vi "to string.vi"(8 "error in":errorcluster, 11 "Modbus Slave configuration in":refnum<class "Modbus Slave configuration.lvclass">) -> (0 "error out":errorcluster, 1 "data":string, 2 "version":string, 3 "Modbus Slave configuration out":refnum<class "Modbus Slave configuration.lvclass">)   [LabVIEW 2013, in "Modbus Slave configuration.lvclass"]
doc: "Provides an interface for saving a module configuration to a file or other serialized data source. It is recommended that all children of this class store data in two sets--data required for its own initialization, and any data required for parent initialization--and that each implementation uses the <b>Call Parent Method</b> primitive to serialize parent information.Platypus Framework 1.0.1.65\nNI Systems Engineering - National Instruments"
uses:
  Modbus Slave configuration.lvclass
  <vilib>/NI/Tag Bus Module Framework/module configuration/TBM module configuration.lvclass
  Modbus Slave configuration.lvclass/Modbus Slave configuration.ctl
  module channel/Modbus Module Channel.lvclass
  <vilib>/NI/Configuration Framework/serializable configuration/NISE_CEF_serializable configuration.lvclass
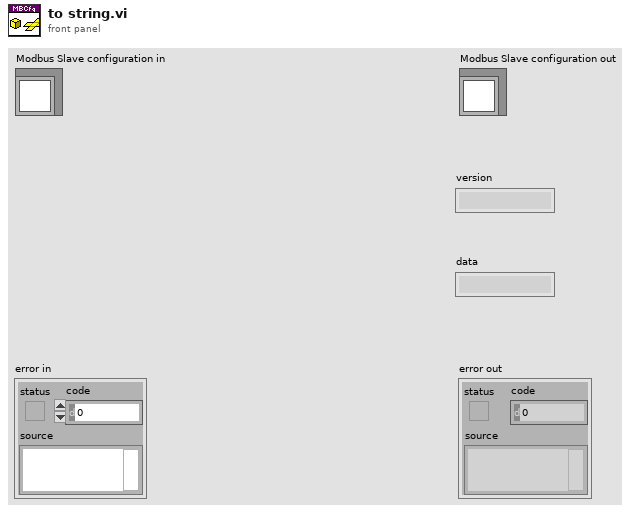
[diagram p1: front panel]
types:
  T1 = typedef "Modbus Slave configuration.lvclass/modbus class.ctl" = enum16{"TCP master", "TCP slave", "serial master", "serial slave"}
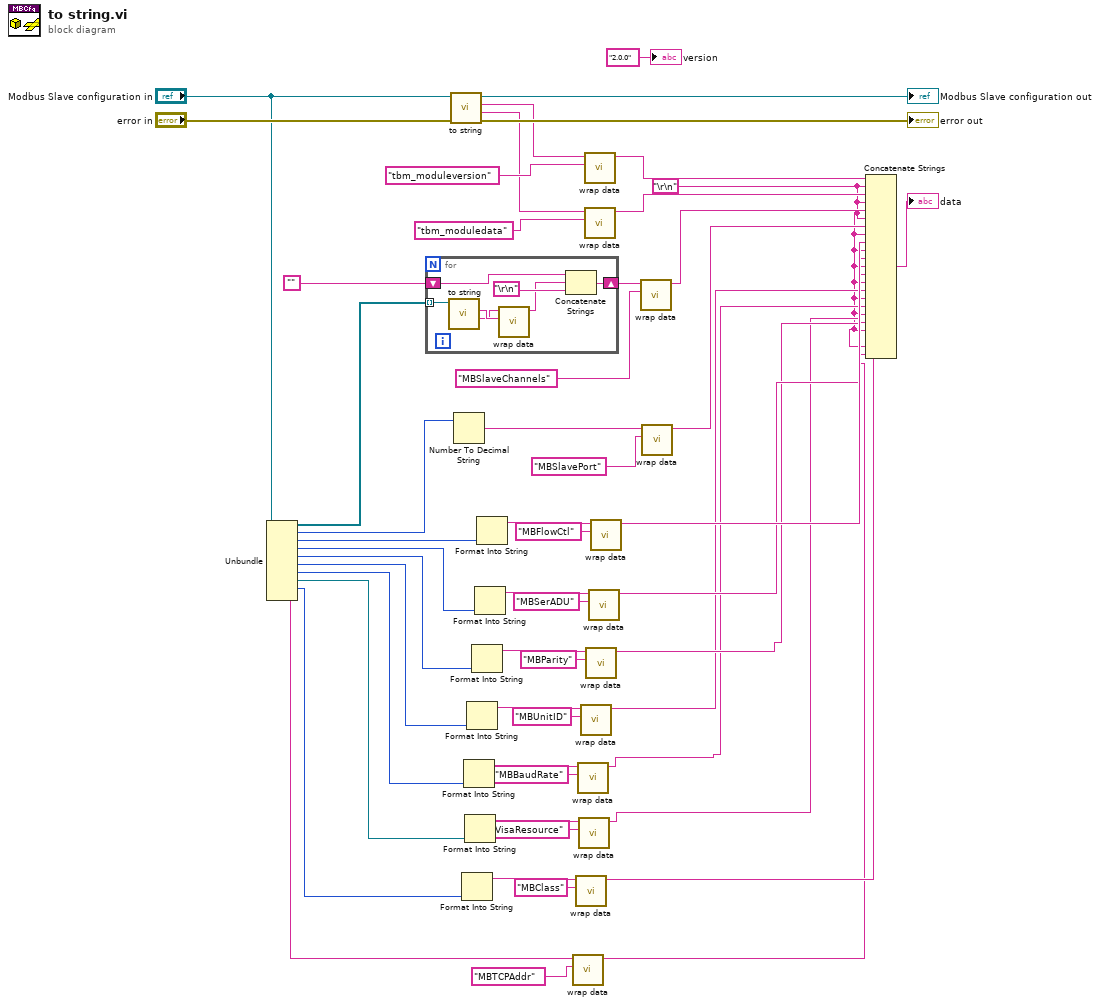
[diagram p0: block diagram]
diagram:
  w4 = "\r\n"
  n1 = Unbundle("Modbus Slave configuration in") -> (w40:refnum<class "Modbus Module Channel.lvclass">[], w35:u16, w31:u16, w17:enum16{"RTU", "ASCII"}, w16:u16, w15:u8, w14:u32, w13:refnum<visa-resource-name>, w12:T1, w3:string)
  n2 = for {
    tunnel: w40 -> [w56] mode=indexing
    shift-right: [w59] -> w38
    shift-left: "" -> [w58]
    n3 = call-dynamic "to string.vi"("channel in"=w56) -> ("channel data"=w54:string, "identifier"=w55:string)  [unwired: 7 in, 2 out]
    n4 = call <vilib>:"wrap data.vi"("identifier"=w55, "data to wrap"=w54) -> ("wrapped data"=w57:string)  [unwired: 9 in]
    n5 = Concatenate Strings(w58, w57, "\r\n") -> (w59:string)
  }
  n6 = call-parent "to string.vi"("error in"="error in", "module configuration in"="Modbus Slave configuration in") -> ("error out"=→"error out":errorcluster, "data"=w45:string, "version"=w46:string, "module configuration out"=→"Modbus Slave configuration out":refnum<class "Modbus Slave configuration.lvclass">)  [unwired: 6 in]
  n7 = Number To Decimal String(number=w35) -> (decimal integer string=w34:string)  [unwired: 1 in]
  n8 = Format Into String(w12) -> (resulting string=w19:string)  [unwired: 3 in, 1 out]
  n9 = Format Into String(w14) -> (resulting string=w24:string)  [unwired: 3 in, 1 out]
  n10 = Format Into String(w13) -> (resulting string=w20:string)  [unwired: 3 in, 1 out]
  n11 = Format Into String(w15) -> (resulting string=w23:string)  [unwired: 3 in, 1 out]
  n12 = Format Into String(w16) -> (resulting string=w27:string)  [unwired: 3 in, 1 out]
  n13 = Format Into String(w17) -> (resulting string=w28:string)  [unwired: 3 in, 1 out]
  n14 = Format Into String(w31) -> (resulting string=w32:string)  [unwired: 3 in, 1 out]
  n15 = call <vilib>:"wrap data.vi"("identifier"="MBTCPAddr", "data to wrap"=w3) -> ("wrapped data"=w2:string)  [unwired: 9 in]
  n16 = call <vilib>:"wrap data.vi"("identifier"="MBClass", "data to wrap"=w19) -> ("wrapped data"=w5:string)  [unwired: 9 in]
  n17 = call <vilib>:"wrap data.vi"("identifier"="MBBaudRate", "data to wrap"=w24) -> ("wrapped data"=w7:string)  [unwired: 9 in]
  n18 = call <vilib>:"wrap data.vi"("identifier"="MBVisaResource", "data to wrap"=w20) -> ("wrapped data"=w6:string)  [unwired: 9 in]
  n19 = call <vilib>:"wrap data.vi"("identifier"="MBUnitID", "data to wrap"=w23) -> ("wrapped data"=w8:string)  [unwired: 9 in]
  n20 = call <vilib>:"wrap data.vi"("identifier"="tbm_moduleversion" ("additional identifier"), "data to wrap"=w46) -> ("wrapped data"=w48:string)  [unwired: 9 in]
  n21 = call <vilib>:"wrap data.vi"("identifier"="tbm_moduledata" ("additional identifier"), "data to wrap"=w45) -> ("wrapped data"=w47:string)  [unwired: 9 in]
  n22 = call <vilib>:"wrap data.vi"("identifier"="MBParity", "data to wrap"=w27) -> ("wrapped data"=w9:string)  [unwired: 9 in]
  n23 = call <vilib>:"wrap data.vi"("identifier"="MBSerADU", "data to wrap"=w28) -> ("wrapped data"=w10:string)  [unwired: 9 in]
  n24 = call <vilib>:"wrap data.vi"("identifier"="MBFlowCtl", "data to wrap"=w32) -> ("wrapped data"=w11:string)  [unwired: 9 in]
  n25 = call <vilib>:"wrap data.vi"("identifier"="MBSlaveChannels" ("additional identifier"), "data to wrap"=w38) -> ("wrapped data"=w42:string)  [unwired: 9 in]
  n26 = call <vilib>:"wrap data.vi"("identifier"="MBSlavePort" ("additional identifier"), "data to wrap"=w34) -> ("wrapped data"=w36:string)  [unwired: 9 in]
  n27 = Concatenate Strings(w48, w4, w47, w4, w42, w4, w36, w4, w11, w4, w10, w4, w9, w4, w8, w4, w7, w4, w6, w4, w5, w4, w2) -> (→"data":string)
  "version" <- "2.0.0" ("current version")
